vi "z-trans test.vi"() -> ()   [LabVIEW 2015]
uses:
  <vilib>/measure/macond.llb/FIR Filter for 1 Chan.vi
  <vilib>/measure/NI_MAPro.lvlib
panel:
  in  "FIR filter specifications":T1={"Topology"=enum."Off", "Type"=enum."Lowpass", "#Taps"=50, "Lower PB"=100.0, "Upper PB"=0.0, "Lower SB"=200.0, "Upper SB"=0.0} {"Lower SB" format="%0.2p"; "Upper SB" format="%0.2p"; "Lower PB" format="%0.2p"; "Upper PB" format="%0.2p"}
  out "Waveform Graph":dbl[][](graph)
  in  "Decimation":i32
  in  "times":i32
  in  "theta":dbl
  out "XY Graph":cluster{dbl[], dbl[]}(graph)
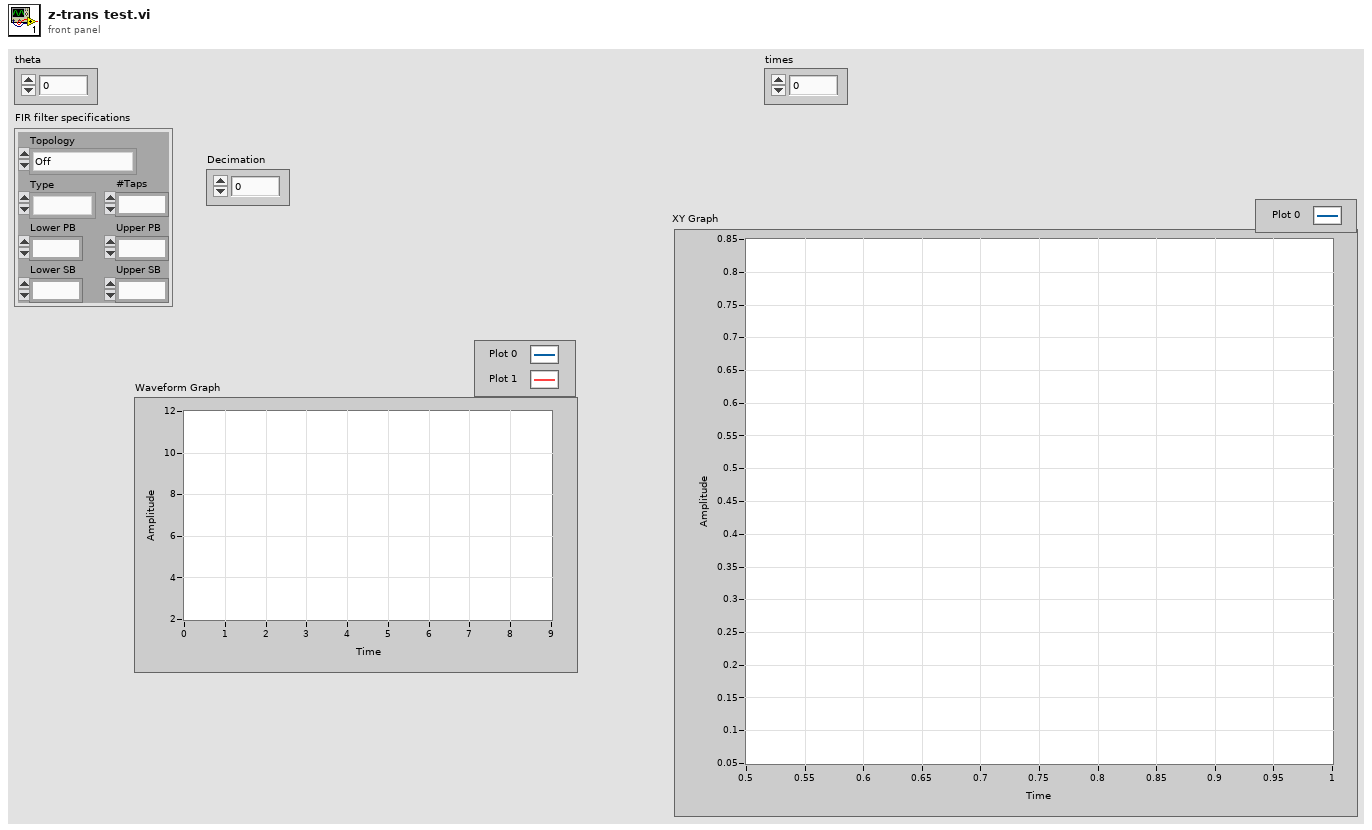
[diagram p1: front panel]
types:
  T1 = cluster{"Topology":enum16{"Off", "FIR by Specification", "Equi-ripple FIR", "Windowed FIR"}, "Type":enum16{"Lowpass", "Highpass", "Bandpass", "Bandstop"}, "#Taps":i32, "Lower PB":dbl, "Upper PB":dbl, "Lower SB":dbl, "Upper SB":dbl}
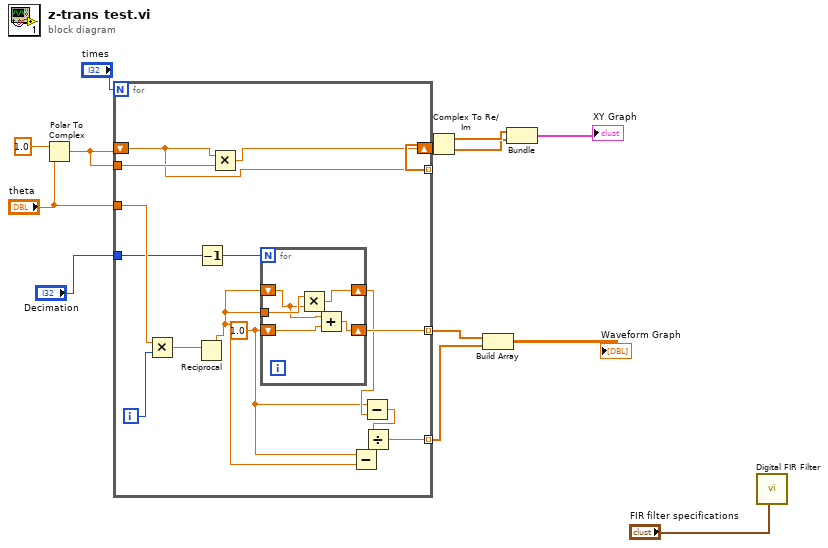
[diagram p0: block diagram]
diagram:
  n1 = Polar To Complex(1:"theta", 2:1.0 ("r")) -> (0:w12:cdb)
  n2 = for {
    N: "times" -> [_]
    shift-right: [w27] -> _
    shift-left: w12 -> [w26]
    tunnel: w12 -> [w28]
    tunnel: [w26] -> w11 mode=indexing
    tunnel: "theta" -> [w24]
    tunnel: "Decimation" -> [w22]
    tunnel: [w21] -> w4 mode=indexing
    tunnel: [w14] -> w2 mode=indexing
    i -> [w25]
    w18 = 1.0
    n3 = Multiply(x=w24, y=w25) -> (x*y=w23:dbl)
    n4 = Reciprocal(x=w23) -> (1/x=w17:dbl)
    n5 = Decrement(x=w22) -> (x-1=w20:i32)
    n6 = Multiply(x=w26, y=w28) -> (x*y=w27:cdb)
    n7 = for {
      N: w20 -> [_]
      shift-right: [w32] -> w19
      shift-left: w17 -> [w30]
      tunnel: w17 -> [w33]
      shift-right: [w31] -> w21
      shift-left: w18 -> [w29]
      n8 = Multiply(x=w33, y=w30) -> (x*y=w32:dbl)
      n9 = Add(x=w30, y=w29) -> (x+y=w31:dbl)
    }
    n10 = Subtract(x=w18, y=w17) -> (x-y=w15:dbl)
    n11 = Subtract(x=w18, y=w19) -> (x-y=w16:dbl)
    n12 = Divide(x=w16, y=w15) -> (x/y=w14:dbl)
  }
  n13 = Complex To Re/Im(x + iy=w11) -> (x=w9:dbl[], y=w8:dbl[])
  n14 = Build Array(w4, w2) -> (→"Waveform Graph":dbl[][])
  n15 = Bundle(w9, w8) -> (→"XY Graph":cluster{dbl[], dbl[]})  [unwired: 1 in]
  n16 = call-poly <vilib>:"Digital FIR Filter.vi"("FIR filter specifications"="FIR filter specifications") -> ()  [unwired: 8 in, 3 out]
